vi "Maestro 6 SCC Servo Example.vi"() -> ()   [LabVIEW 2018]
uses:
  <vilib>/Instr/_visa.llb/VISA Configure Serial Port (Instr).vi
  <vilib>/Utility/inputDevices.llb/joystickAcquire.vi
  <vilib>/Utility/inputDevices.llb/closeJoystick.vi
  <vilib>/ptbypt/NI_PtbyPt.lvlib
panel:
  in  "OK Button":bool
  out "Lap Times":dbl[](array[numeric])
  in  "device index 2":i32=2
  out "Elapsed Time (s)":dbl=6.446096897125244
  out "X Axis 4":i32=128
  out "X Axis 3":i32=128
  out "X Axis 2":i32=128
  out "X Axis":i32=128
  out "axis info":T1={"X axis"=-2, "Y axis"=-2, "Z axis"=-2, "X axis rotation"=-2, "Y axis rotation"=-2, "Z axis rotation"=-2, "U axis"=-2, "V axis"=-2}
  in  "device index":i32
  in  "stop":bool
  # "Pololu Maestro 6"
  # "SSC Servo \nControl Example"
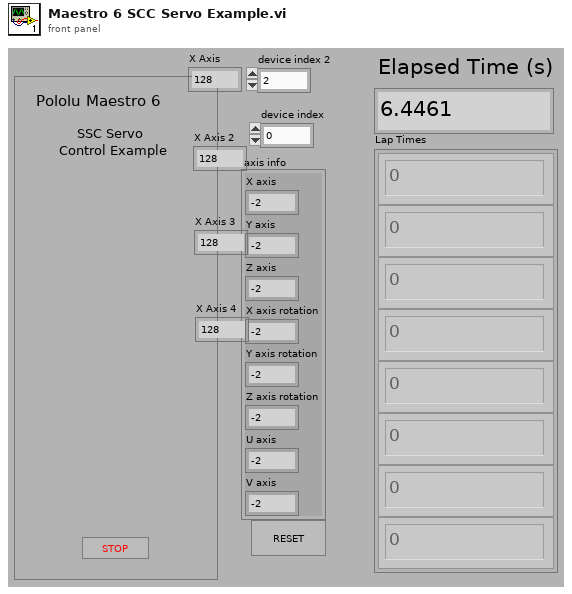
[diagram p1: front panel]
types:
  T1 = cluster{"X axis":i32, "Y axis":i32, "Z axis":i32, "X axis rotation":i32, "Y axis rotation":i32, "Z axis rotation":i32, "U axis":i32, "V axis":i32}
  T2 = cluster{"button 1":bool, "button 2":bool, "button 3":bool, "button 4":bool, "button 5":bool, "button 6":bool, "button 7":bool, "button 8":bool, "button 9":bool, "button 10":bool, "button 11":bool, "button 12":bool, "button 13":bool, "button 14":bool, "button 15":bool, "button 16":bool, "button 17":bool, "button 18":bool, "button 19":bool, "button 20":bool, "button 21":bool, "button 22":bool, "button 23":bool, "button 24":bool, "button 25":bool, "button 26":bool, "button 27":bool, "button 28":bool, "button 29":bool, "button 30":bool, "button 31":bool, "button 32":bool}
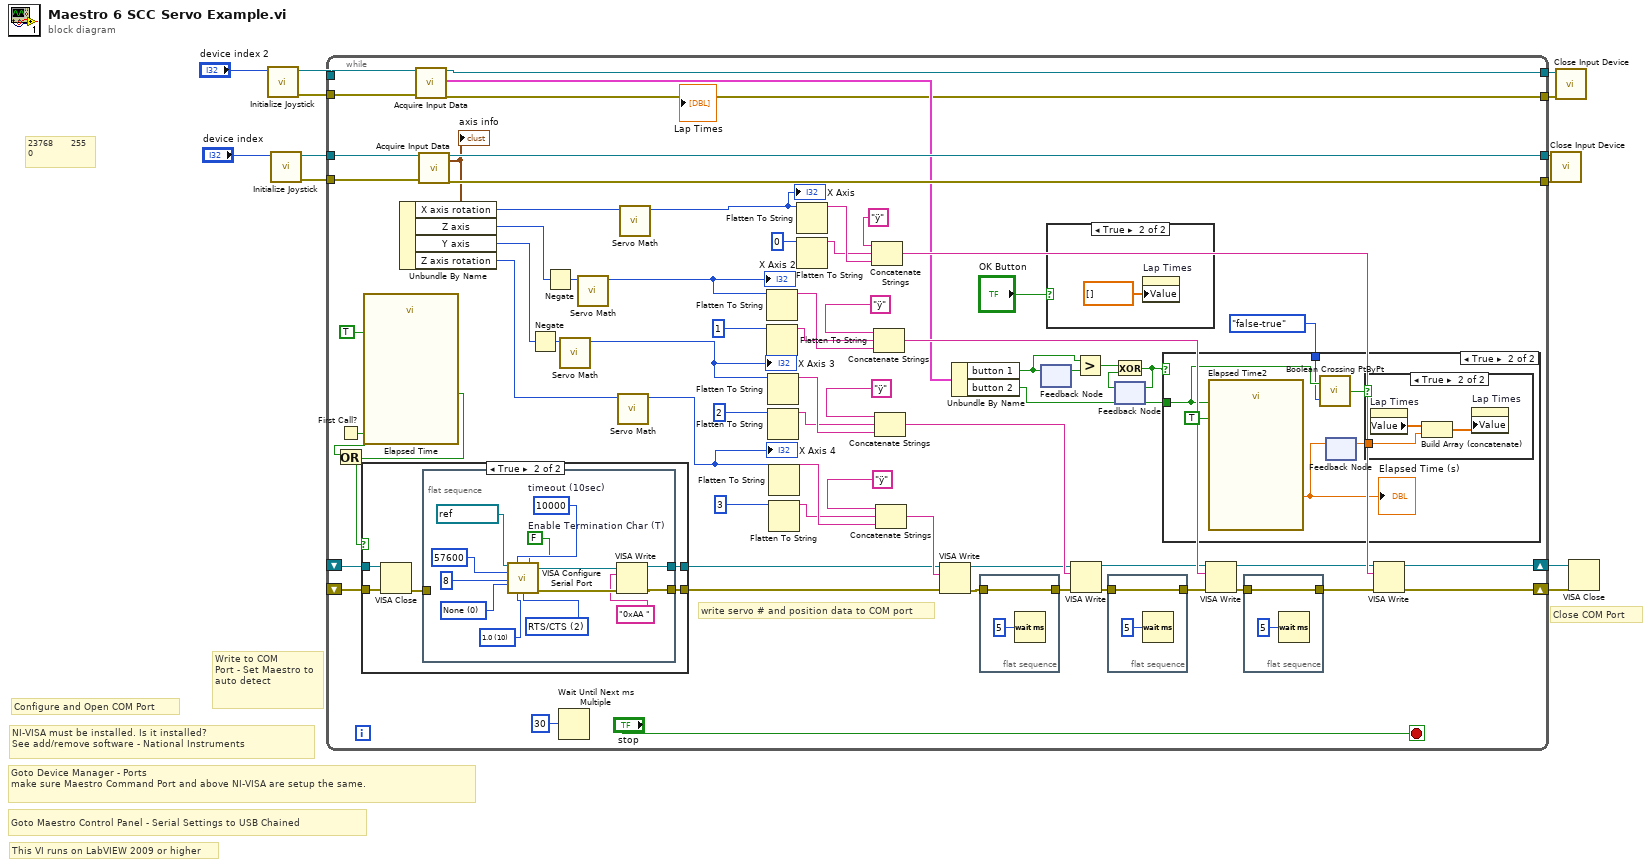
[diagram p0: block diagram]
diagram:
  # "23768      255\n0"
  # "This VI runs on LabVIEW 2009 or higher"
  # "Goto Maestro Control Panel - Serial Settings to USB Chained"
  # "Close COM Port"
  # "Configure and Open COM Port"
  # "Goto Device Manager - Ports \nmake sure Maestro Command Port and above NI-VISA are setup the same."
  # "NI-VISA must be installed. Is it installed?\nSee add/remove software - National Instruments"
  # "Write to COM \nPort - Set Maestro to auto detect"
  n1 = call <vilib>:"Initialize Joystick.vi"("device index"="device index 2") -> ("error out"=w5:errorcluster, "device ID"=w4:refnum<k1>)  [unwired: 9 in]
  n2 = call <vilib>:"Initialize Joystick.vi"("device index"="device index") -> ("error out"=w8:errorcluster, "device ID"=w9:refnum<k1>)  [unwired: 9 in]
  n3 = while {
    tunnel: w9 -> [w75]
    tunnel: w8 -> [w74]
    tunnel: [w73] -> w7
    tunnel: [w72] -> w6
    shift-right: [w76] -> w11
    shift-left: _ -> [w36]
    shift-right: [w77] -> w12
    shift-left: _ -> [w37]
    tunnel: w4 -> [w18]
    tunnel: w5 -> [w19]
    tunnel: [w16] -> w2
    tunnel: [w15] -> w1
    stop <- "stop" stop-if-true
    # "write servo # and position data to COM port"
    n4 = First Call?() -> (First Call?: T/F=w26:bool)
    n5 = call "Elapsed Time"("Auto Reset"=TRUE) -> ("Time has Elapsed"=w35:bool)  [unwired: 11 in, 7 out]
    n6 = Or(x=w26, y=w35) -> (x .or. y?=w33:bool)
    n7 = case shown="True" w33 {
      tunnel: [w99 w104] -> w39
      tunnel: [w98 w103] -> w38
      tunnel: w37 -> [w99 w102]
      tunnel: w36 -> [w98 w101]
      frame False {
      }
      frame True {
        n8 = VISA Close(VISA resource name=w102, error in (no error)=w101) -> (error out=w100:errorcluster)
        n9 = flat-sequence {
          tunnel: [w106] -> w104
          tunnel: [w105] -> w103
          tunnel: w100 -> [_]
          frame #0 {
            w108 = u16 2 items=["None"=0, "XON/XOFF"=1, "RTS/CTS"=2, "DTR/DSR"=4] ("flow control")
            w109 = u16 10 items=["1.0"=10, "1.5"=15, "2.0"=20] ("stop bits")
            w110 = u16 0 items=["None", "Odd", "Even", "Mark", "Space"] ("parity")
            w113 = FALSE  # Enable Termination Char (T)
            w114 = u32 10000  # timeout (10sec)
            n10 = call-poly "VISA Configure Serial Port"("VISA resource name"=refnum<visa-resource-name> "COM6", "timeout (10sec)"=w114, "Enable Termination\nChar (T)"=w113, "baud rate (9600)"=u32 57600 ("baud rate"), "data bits (8)"=u16 8 ("data bits"), "parity (0:none)"=w110, "stop bits (10: 1 bit)"=w109, "flow control (0:none)"=w108) -> ("VISA resource name out"=w117:refnum<visa-resource-name>, "error out"=w116:errorcluster)  [unwired: 1 in, 5 out]
            n11 = VISA Write(VISA resource name=w117, write buffer="0xAA ", error in (no error)=w116) -> (VISA resource name out=w106:refnum<visa-resource-name>, error out=w105:errorcluster)  [unwired: 1 out]
          }
        }
      }
    }
    n12 = call-poly <vilib>:"Acquire Input Data.vi"("device ID"=w18, "error in (no error)"=w19) -> ("device ID"=w16:refnum<k1>, "button info"=w17:T2, "error out"=w15:errorcluster)  [unwired: 13 in, 2 out]
    n13 = call-poly <vilib>:"Acquire Input Data.vi"("device ID"=w75, "error in (no error)"=w74) -> ("device ID"=w73:refnum<k1>, "axis info"=w71:T1, "error out"=w72:errorcluster)  [unwired: 13 in, 2 out]
    "axis info" <- w71
    n14 = Unbundle By Name(w71) -> ("X axis rotation"=w51:i32, "Z axis"=w49:i32, "Y axis"=w47:i32, "Z axis rotation"=w45:i32)
    n15 = Negate(x=w47) -> (-x=w40:i32)
    n16 = Negate(x=w49) -> (-x=w41:i32)
    n17 = Wait Until Next ms Multiple(millisecond multiple=30) -> ()  [unwired: 1 out]
    n18 = call "Servo Math.vi"("X axis rotation"=w40) -> ("Numeric"=w46:u8)  [unwired: 10 in]
    "X Axis 3" <- w46
    n19 = call "Servo Math.vi"("X axis rotation"=w41) -> ("Numeric"=w48:u8)  [unwired: 10 in]
    "X Axis 2" <- w48
    n20 = call "Servo Math.vi"("X axis rotation"=w45) -> ("Numeric"=w44:u8)  [unwired: 10 in]
    "X Axis 4" <- w44
    n21 = call "Servo Math.vi"("X axis rotation"=w51) -> ("Numeric"=w50:u8)  [unwired: 10 in]
    "X Axis" <- w50
    n22 = Flatten To String(anything=w48) -> (data string=w57:string)  [unwired: 1 in, 4 out]
    n23 = Flatten To String(anything=u8 1 ("position")) -> (data string=w56:string)  [unwired: 1 in, 4 out]
    n24 = Flatten To String(anything=w46) -> (data string=w55:string)  [unwired: 1 in, 4 out]
    n25 = Flatten To String(anything=u8 2 ("position")) -> (data string=w54:string)  [unwired: 1 in, 4 out]
    n26 = Flatten To String(anything=w44) -> (data string=w53:string)  [unwired: 1 in, 4 out]
    n27 = Flatten To String(anything=u8 3 ("position")) -> (data string=w52:string)  [unwired: 1 in, 4 out]
    n28 = Flatten To String(anything=w50) -> (data string=w59:string)  [unwired: 1 in, 4 out]
    n29 = Flatten To String(anything=u8 0 ("position")) -> (data string=w58:string)  [unwired: 1 in, 4 out]
    n30 = Concatenate Strings("ÿ", w58, w59) -> (w61:string)
    n31 = Concatenate Strings("ÿ", w56, w57) -> (w62:string)
    n32 = Concatenate Strings("ÿ", w54, w55) -> (w63:string)
    n33 = Concatenate Strings("ÿ", w52, w53) -> (w64:string)
    n34 = VISA Write(VISA resource name=w39, write buffer=w64, error in (no error)=w38) -> (VISA resource name out=w43:refnum<visa-resource-name>, error out=w31:errorcluster)  [unwired: 1 out]
    n35 = Unbundle By Name(w17) -> ("button 1"=w23:bool, "button 2"=w25:bool)
    n36 = flat-sequence {
      tunnel: [w97] -> w32
      tunnel: w31 -> [w97]
      frame #0 {
        n37 = Wait (ms)(milliseconds to wait=u32 5) -> ()  [unwired: 1 out]
      }
    }
    n38 = feedback-in #1(w23) -> ()
    n39 = feedback #1() -> (w24:bool)  [unwired: 1 in]
    n40 = case shown="True" "OK Button" {
      frame False {
      }
      frame True {
        n41 = property on="Lap Times" class="Arr (strict)"("Value"=dbl[] [] ("Lap Times")) -> ()  [unwired: 2 in, 2 out]
      }
    }
    n42 = VISA Write(VISA resource name=w43, write buffer=w63, error in (no error)=w32) -> (VISA resource name out=w42:refnum<visa-resource-name>, error out=w30:errorcluster)  [unwired: 1 out]
    n43 = Greater?(x=w23, y=w24) -> (0:w22:bool)
    n44 = flat-sequence {
      tunnel: [w95] -> w29
      tunnel: w30 -> [w95]
      frame #0 {
        n45 = Wait (ms)(milliseconds to wait=u32 5) -> ()  [unwired: 1 out]
      }
    }
    n46 = feedback #2() -> (w21:bool)  [unwired: 1 in]
    n47 = Exclusive Or(1:w21, 2:w22) -> (0:w20:bool)
    n48 = feedback-in #2(w20) -> ()
    n49 = case shown="True" w20 {
      tunnel: w25 -> [_ w87]
      tunnel: enum16{"either", "false-true", "true-false"}."false-true" ("direction") -> [_ w85]
      frame False {
      }
      frame True {
        n50 = call "Elapsed Time2"("Reset"=w87, "Auto Reset"=TRUE) -> ("Elapsed Time (s)"=w84:dbl)  [unwired: 10 in, 7 out]
        "Elapsed Time (s)" <- w84
        n51 = call <vilib>:"Boolean Crossing PtByPt.vi"("direction"=w85, "input"=w87) -> ("crossing"=w86:bool)  [unwired: 1 in]
        n52 = feedback #3() -> (w83:dbl)  [unwired: 1 in]
        n53 = feedback-in #3(w84) -> ()
        n54 = case shown="True" w86 {
          tunnel: w83 -> [_ w89]
          frame False {
          }
          frame True {
            n55 = property on="Lap Times" class="Arr (strict)"() -> ("Value"=w90:dbl[])  [unwired: 2 in, 2 out]
            n56 = Build Array (concatenate)(w90, w89) -> (w91:dbl[])
            n57 = property on="Lap Times" class="Arr (strict)"("Value"=w91) -> ()  [unwired: 2 in, 2 out]
          }
        }
      }
    }
    n58 = VISA Write(VISA resource name=w42, write buffer=w62, error in (no error)=w29) -> (VISA resource name out=w60:refnum<visa-resource-name>, error out=w28:errorcluster)  [unwired: 1 out]
    n59 = flat-sequence {
      tunnel: [w93] -> w27
      tunnel: w28 -> [w93]
      frame #0 {
        n60 = Wait (ms)(milliseconds to wait=u32 5) -> ()  [unwired: 1 out]
      }
    }
    n61 = VISA Write(VISA resource name=w60, write buffer=w61, error in (no error)=w27) -> (VISA resource name out=w77:refnum<visa-resource-name>, error out=w76:errorcluster)  [unwired: 1 out]
  }
  n62 = call-poly <vilib>:"Close Input Device.vi"("error in (no error)"=w6, "device ID"=w7) -> ()  [unwired: 8 in, 1 out]
  n63 = call-poly <vilib>:"Close Input Device.vi"("error in (no error)"=w1, "device ID"=w2) -> ()  [unwired: 8 in, 1 out]
  n64 = VISA Close(VISA resource name=w12, error in (no error)=w11) -> ()  [unwired: 1 out]
